vi "Read Attribute Meta Data.vi"(7 "Linked List ID":string, 8 "error in (no error)":errorcluster, 9 "Attribute Type":variant, 10 "Attribute Name":string, 11 "Linked List in":refnum<class "Linked List.lvclass">) -> (0 "error out":errorcluster, 1 "Found?":bool, 2 "Meta Data":string, 3 "Linked List out":refnum<class "Linked List.lvclass">)   [LabVIEW 2020, in "Linked Lists.lvlib" / "Linked List.lvclass"]
uses:
  <vilib>/gpm_packages/@cs/linked-list/Source/Linked List/Linked List/Linked List.lvclass
  <vilib>/gpm_packages/@cs/linked-list/Source/Linked List/Linked List/Linked List.lvclass/Linked List.ctl
  <vilib>/gpm_packages/@cs/lookup-table/Source/LookupTable/LookupTable.lvclass/LookupTable.ctl
  9a566823-d82a-4411-bf8b-9d15e8d92693.vi
  <vilib>/gpm_packages/@cs/lookup-table/Source/LookupTable/Read Table Reference.vi
  9a566823-d82a-4411-bf8b-9d15e8d92693.vi/fbe630d9-a52d-48cb-9360-ee4309b2b274.vi
  <vilib>/gpm_packages/@cs/lookup-table/Source/LookupTable/LookupTable.lvclass
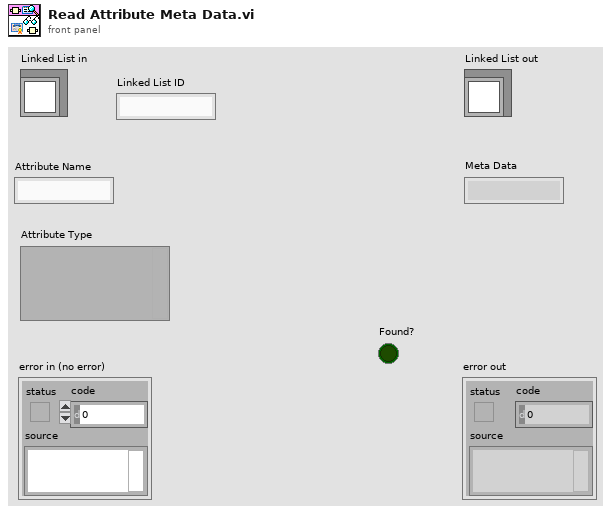
[diagram p1: front panel]
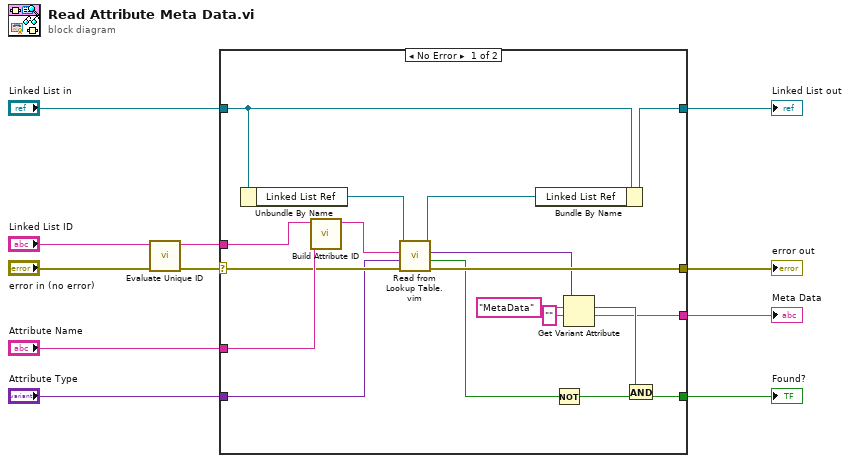
[diagram p0: block diagram]
diagram:
  n1 = call <vilib>:"Evaluate Unique ID.vi"("error in (no error)"="error in (no error)", "Unique ID"="Linked List ID") -> ("error out"=w9:errorcluster, "Unique ID Out"=w8:string)  [unwired: 8 in]
  n2 = case shown="No Error" w9 {
    selector: w9 -> [w25 w30]
    tunnel: w8 -> [w27 _]
    tunnel: "Linked List in" -> [w26 w31]
    tunnel: [w28 w31] -> w6
    tunnel: "Attribute Name" -> [w29 _]
    tunnel: "Attribute Type" -> [w20 _]
    tunnel: [w24 w30] -> w3
    tunnel: [w14 _] -> w2
    tunnel: [w12 _] -> w1
    frame No Error {
      n3 = Unbundle By Name(w26) -> ("Linked List Ref"=w23:refnum<data-value>)
      n4 = call <vilib>:"Build Attribute ID.vi"("Attr Name"=w29, "Unique ID"=w27) -> ("Attr ID Out"=w21:string)  [unwired: 9 in]
      n5 = call "Read from Lookup Table.vim"("error in (no error)"=w25, "Type"=w20, "Item Name"=w21, "LookupTable Reference"=w23) -> ("error out"=w24:errorcluster, "Not Found?"=w19:bool, "Value"=w17:variant, "LookupTable Reference Out"=w22:refnum<data-value>)  [unwired: 4 in]
      n6 = Bundle By Name(cluster=w26, "Linked List Ref"=w22) -> (w28:refnum<class "Linked List.lvclass">)
      n7 = Not(x=w19) -> (.not. x?=w18:bool)
      n8 = Get Variant Attribute(Variant=w17, name="MetaData", default value (empty Variant)="") -> (found=w13:bool, value=w12:string)  [unwired: 1 in, 2 out]
      n9 = And(x=w13, y=w18) -> (x .and. y?=w14:bool)
    }
    frame Error {
    }
  }
  "error out" <- w3
  "Linked List out" <- w6
  "Meta Data" <- w1
  "Found?" <- w2
